vi "Logical Channel.vi"(8 "error in (no error)":errorcluster, 10 "12 Logicals inputs state":T1[](array[typedef]) items=["Off", "On", "Ignore"], 11 "VISA resource name":refnum<visa-resource-name>) -> (0 "error out":errorcluster, 3 "VISA resource name out":refnum<visa-resource-name>)   [LabVIEW 2017, in "Sefram DAS220.lvlib"]
doc: "Trig on logical mask according to the 12 digital channels states."
uses:
  <instrlib>/Sefram DAS220/Sefram DAS220.lvlib
  <instrlib>/Sefram DAS220/Public/Configure/Triggers-Alarms/Low-level/Trigger Types/Logical TriState.ctl
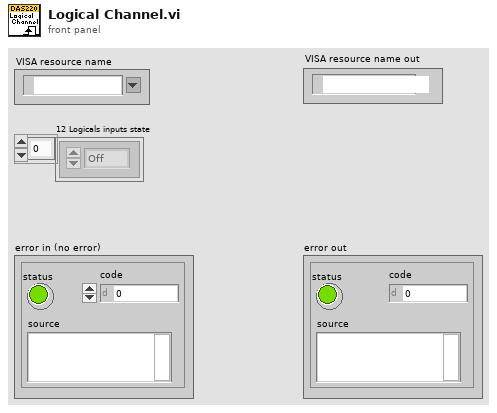
[diagram p1: front panel]
types:
  T1 = typedef "Sefram DAS220.lvlib/Logical TriState.ctl" = u16
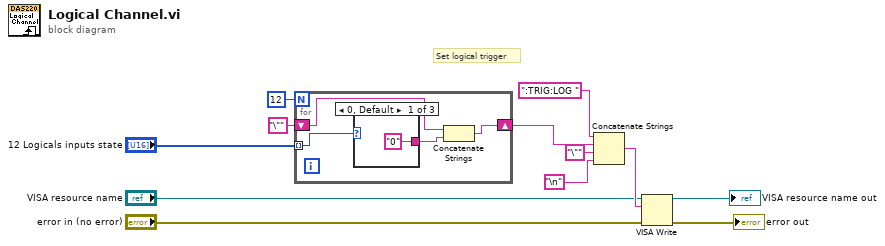
[diagram p0: block diagram]
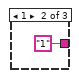
[diagram p2: hidden frame]
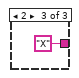
[diagram p3: hidden frame]
diagram:
  # "Set logical trigger"
  n1 = for {
    N: 12 -> [_]
    tunnel: "12 Logicals inputs state" -> [w16] mode=indexing
    shift-right: [w13] -> w3
    shift-left: "\"" -> [w14]
    n2 = case shown="0, Default" w16 {
      tunnel: ["0" "1" "X"] -> w15
      frame 0, Default {
      }
      frame 1 {
      }
      frame 2 {
      }
    }
    n3 = Concatenate Strings(w14, w15) -> (w13:string)
  }
  n4 = Concatenate Strings(":TRIG:LOG " ("string"), w3, "\"" ("string"), "\n") -> (w12:string)
  n5 = VISA Write(VISA resource name="VISA resource name", write buffer=w12, error in (no error)="error in (no error)") -> (VISA resource name out=→"VISA resource name out":refnum<visa-resource-name>, error out=→"error out":errorcluster)  [unwired: 1 out]
